vi "Review Result.vi"(0 "Path in":refnum<class "Path.lvclass">, 11 "error in (no error)":errorcluster) -> (4 "Path out":refnum<class "Path.lvclass">, 6 "Response":string, 15 "error out":errorcluster)   [LabVIEW 2023, in "RFCalAndFixtureCharact.Common.lvlib" / "Path.lvclass"]
uses:
  Path.lvclass
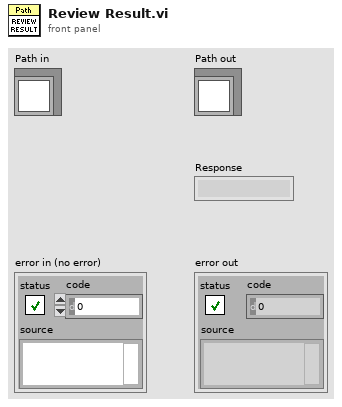
[diagram p1: front panel]
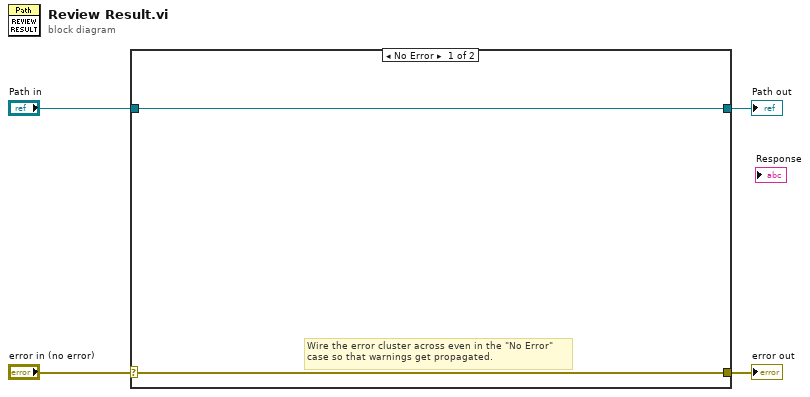
[diagram p0: block diagram]
diagram:
  n1 = case shown="No Error" "error in (no error)" {
    selector: "error in (no error)" -> [w5 w8]
    tunnel: [w5 w8] -> w3
    tunnel: [w6 w7] -> w1
    tunnel: "Path in" -> [w6 w7]
    frame No Error {
      # "Wire the error cluster across even in the \"No Error\"\ncase so that warnings get propagated."
    }
    frame Error {
    }
  }
  "error out" <- w3
  "Path out" <- w1
